vi "draw enemies.vi"(0 "Array of rows for every enemy":dbl[](array[numeric]), 1 "enemies on board":dbl[](array[numeric]), 2 "number of enemies":i32, 5 "big rock":u32[][](array[numeric]), 7 "array of columns for every enemy":dbl[](array[numeric]), 9 "rock":u32[][](array[numeric]), 12 "blank Board in":u32[][](array[numeric]), 13 "UFO Ship":u32[][](array[numeric]), 14 "small rock":u32[][](array[numeric])) -> (4 "Board with enemies out":u32[][](array[numeric]))   [LabVIEW 2019]
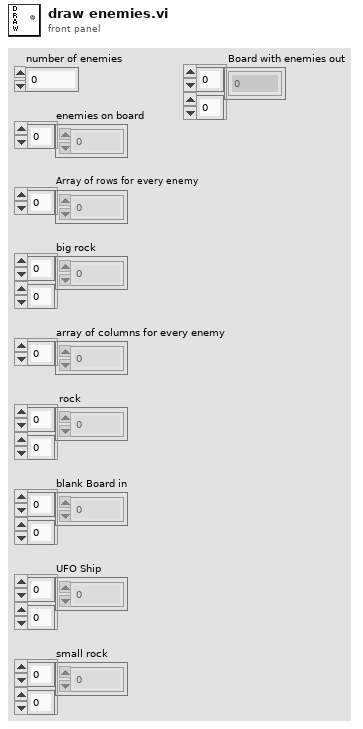
[diagram p1: front panel]
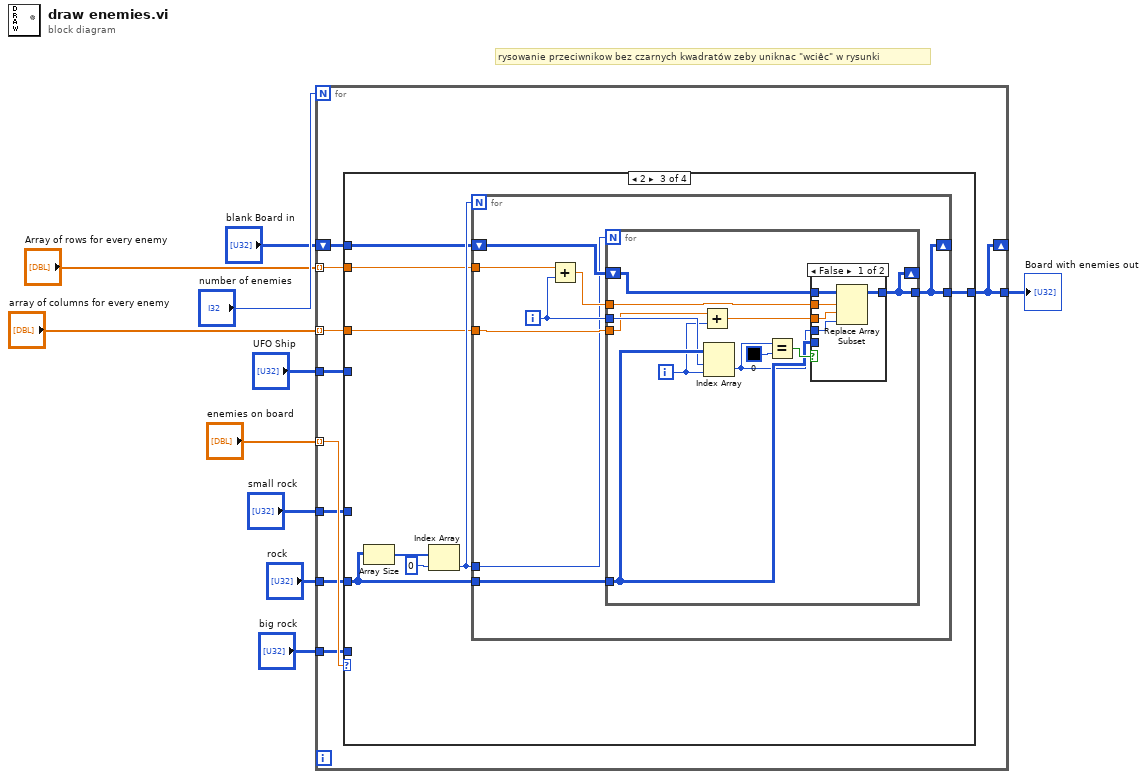
[diagram p0: block diagram]
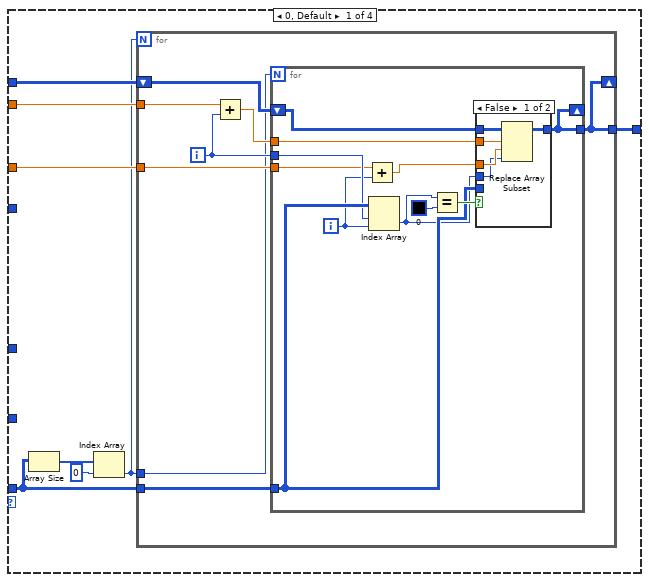
[diagram p2: hidden frame]
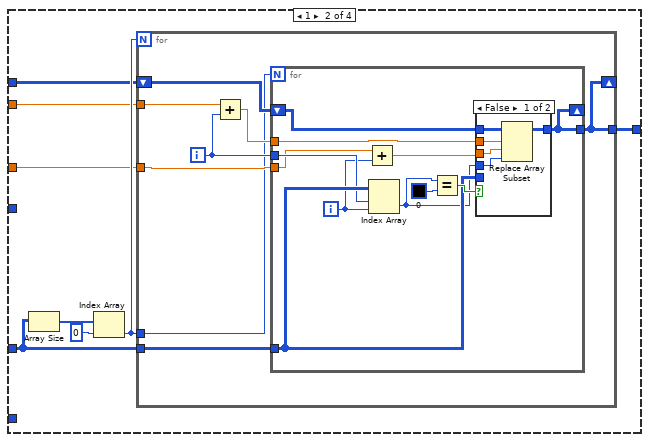
[diagram p4: hidden frame]
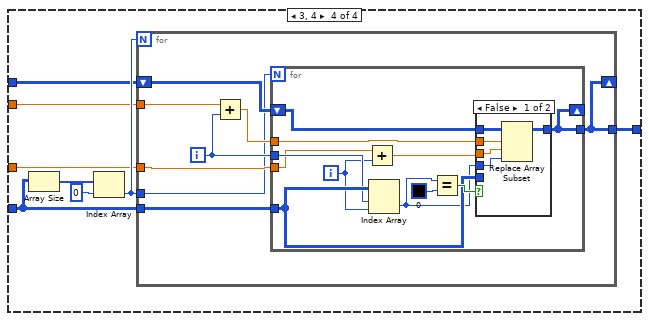
[diagram p7: hidden frame]
diagram:
  # "rysowanie przeciwnikow bez czarnych kwadratów zeby uniknac \"wciêc\" w rysunki"
  n1 = for {
    N: "number of enemies" -> [_]
    tunnel: [w18] -> w1
    tunnel: "enemies on board" -> [w17] mode=indexing
    shift-right: [w18] -> _
    shift-left: "blank Board in" -> [w19]
    tunnel: "Array of rows for every enemy" -> [w15] mode=indexing
    tunnel: "array of columns for every enemy" -> [w16] mode=indexing
    tunnel: "UFO Ship" -> [w14]
    tunnel: "small rock" -> [w13]
    tunnel: "rock" -> [w12]
    tunnel: "big rock" -> [w11]
    n2 = case shown="2" w17 {
      tunnel: w12 -> [_ _ w89 _]
      tunnel: w14 -> [_ _ _ w122]
      tunnel: w13 -> [_ w56 _ _]
      tunnel: w11 -> [w23 _ _ _]
      tunnel: w19 -> [w24 w53 w86 w119]
      tunnel: [w25 w57 w90 w123] -> w18
      tunnel: w15 -> [w27 w54 w87 w120]
      tunnel: w16 -> [w26 w55 w88 w121]
      frame 0, Default {
        n3 = Array Size(array=w23) -> (size(s)=w22:i32[])
        n4 = Index Array(array=w22, index=0) -> (element=w20:i32)
        n5 = for {
          N: w20 -> [_]
          tunnel: w23 -> [w35]
          tunnel: w27 -> [w31]
          tunnel: w26 -> [w34]
          shift-right: [w32] -> _
          shift-left: w24 -> [w33]
          tunnel: [w32] -> w25
          tunnel: w20 -> [w28]
          i -> [w30]
          n6 = Add(x=w31, y=w30) -> (x+y=w29:dbl)
          n7 = for {
            N: w28 -> [_]
            tunnel: w35 -> [w43]
            tunnel: w29 -> [w44]
            tunnel: w34 -> [w38]
            shift-right: [w40] -> _
            shift-left: w33 -> [w42]
            tunnel: [w40] -> w32
            tunnel: w30 -> [w39]
            i -> [w36]
            n8 = Add(x=w38, y=w36) -> (x+y=w37:dbl)
            n9 = Index Array(array=w43, index (row)=w39, index (col)=w36) -> (element=w41:u32)
            n10 = Equal?(x=w41, y=u32 0 ("Color Box")) -> (x = y?=w45:bool)
            n11 = case shown="False" w45 {
              tunnel: w43 -> [_ _]
              tunnel: w44 -> [w51 _]
              tunnel: w37 -> [w50 _]
              tunnel: w42 -> [w48 w52]
              tunnel: [w47 w52] -> w40
              tunnel: w41 -> [w49 _]
              frame False {
                n12 = Replace Array Subset(array=w48, new element=w49, index (row)=w51, index (col)=w50) -> (w47:u32[][])
              }
              frame True {
              }
            }
          }
        }
      }
      frame 1 {
        n13 = Array Size(array=w56) -> (size(s)=w60:i32[])
        n14 = Index Array(array=w60, index=0) -> (element=w58:i32)
        n15 = for {
          N: w58 -> [_]
          tunnel: w56 -> [w68]
          tunnel: w54 -> [w64]
          tunnel: w55 -> [w67]
          shift-right: [w65] -> _
          shift-left: w53 -> [w66]
          tunnel: [w65] -> w57
          tunnel: w58 -> [w61]
          i -> [w63]
          n16 = Add(x=w64, y=w63) -> (x+y=w62:dbl)
          n17 = for {
            N: w61 -> [_]
            tunnel: w68 -> [w76]
            tunnel: w62 -> [w77]
            tunnel: w67 -> [w71]
            shift-right: [w73] -> _
            shift-left: w66 -> [w75]
            tunnel: [w73] -> w65
            tunnel: w63 -> [w72]
            i -> [w69]
            n18 = Add(x=w71, y=w69) -> (x+y=w70:dbl)
            n19 = Index Array(array=w76, index (row)=w72, index (col)=w69) -> (element=w74:u32)
            n20 = Equal?(x=w74, y=u32 0 ("Color Box")) -> (x = y?=w78:bool)
            n21 = case shown="False" w78 {
              tunnel: w76 -> [_ _]
              tunnel: w77 -> [w84 _]
              tunnel: w70 -> [w83 _]
              tunnel: w75 -> [w81 w85]
              tunnel: [w80 w85] -> w73
              tunnel: w74 -> [w82 _]
              frame False {
                n22 = Replace Array Subset(array=w81, new element=w82, index (row)=w84, index (col)=w83) -> (w80:u32[][])
              }
              frame True {
              }
            }
          }
        }
      }
      frame 2 {
        n23 = Array Size(array=w89) -> (size(s)=w93:i32[])
        n24 = Index Array(array=w93, index=0) -> (element=w91:i32)
        n25 = for {
          N: w91 -> [_]
          tunnel: w89 -> [w101]
          tunnel: w87 -> [w97]
          tunnel: w88 -> [w100]
          shift-right: [w98] -> _
          shift-left: w86 -> [w99]
          tunnel: [w98] -> w90
          tunnel: w91 -> [w94]
          i -> [w96]
          n26 = Add(x=w97, y=w96) -> (x+y=w95:dbl)
          n27 = for {
            N: w94 -> [_]
            tunnel: w101 -> [w109]
            tunnel: w95 -> [w110]
            tunnel: w100 -> [w104]
            shift-right: [w106] -> _
            shift-left: w99 -> [w108]
            tunnel: [w106] -> w98
            tunnel: w96 -> [w105]
            i -> [w102]
            n28 = Add(x=w104, y=w102) -> (x+y=w103:dbl)
            n29 = Index Array(array=w109, index (row)=w105, index (col)=w102) -> (element=w107:u32)
            n30 = Equal?(x=w107, y=u32 0 ("Color Box")) -> (x = y?=w111:bool)
            n31 = case shown="False" w111 {
              tunnel: w109 -> [_ _]
              tunnel: w110 -> [w117 _]
              tunnel: w103 -> [w116 _]
              tunnel: w108 -> [w114 w118]
              tunnel: [w113 w118] -> w106
              tunnel: w107 -> [w115 _]
              frame False {
                n32 = Replace Array Subset(array=w114, new element=w115, index (row)=w117, index (col)=w116) -> (w113:u32[][])
              }
              frame True {
              }
            }
          }
        }
      }
      frame 3, 4 {
        n33 = Array Size(array=w122) -> (size(s)=w126:i32[])
        n34 = Index Array(array=w126, index=0) -> (element=w124:i32)
        n35 = for {
          N: w124 -> [_]
          tunnel: w122 -> [w134]
          tunnel: w120 -> [w130]
          tunnel: w121 -> [w133]
          shift-right: [w131] -> _
          shift-left: w119 -> [w132]
          tunnel: [w131] -> w123
          tunnel: w124 -> [w127]
          i -> [w129]
          n36 = Add(x=w130, y=w129) -> (x+y=w128:dbl)
          n37 = for {
            N: w127 -> [_]
            tunnel: w134 -> [w142]
            tunnel: w128 -> [w143]
            tunnel: w133 -> [w137]
            shift-right: [w139] -> _
            shift-left: w132 -> [w141]
            tunnel: [w139] -> w131
            tunnel: w129 -> [w138]
            i -> [w135]
            n38 = Add(x=w137, y=w135) -> (x+y=w136:dbl)
            n39 = Index Array(array=w142, index (row)=w138, index (col)=w135) -> (element=w140:u32)
            n40 = Equal?(x=w140, y=u32 0 ("Color Box")) -> (x = y?=w144:bool)
            n41 = case shown="False" w144 {
              tunnel: w142 -> [_ _]
              tunnel: w143 -> [w150 _]
              tunnel: w136 -> [w149 _]
              tunnel: w141 -> [w147 w151]
              tunnel: [w146 w151] -> w139
              tunnel: w140 -> [w148 _]
              frame False {
                n42 = Replace Array Subset(array=w147, new element=w148, index (row)=w150, index (col)=w149) -> (w146:u32[][])
              }
              frame True {
              }
            }
          }
        }
      }
    }
  }
  "Board with enemies out" <- w1
